vi "ForceBreakPt.vi"(2 "error in":errorcluster, 3 "Bd ID in":u8=1) -> (0 "error out":errorcluster, 1 "Bd ID Out":u8=1)   [LabVIEW 2022 SP3]
uses:
  <vilib>/Motion/FlexMotion/FunctionsVIs/MotionIO.llb/Set Breakpoint Output MOMO (8 axes).flx
  <vilib>/Motion/FlexMotion/CustomControls/CustomControls.llb/Mask (8 axes).flx
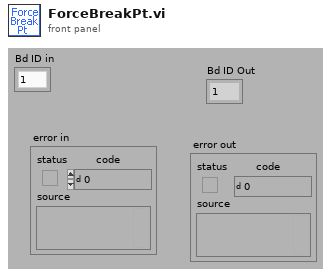
[diagram p1: front panel]
types:
  T1 = typedef "Mask (8 axes).flx" = cluster{"1":bool, "2":bool, "3":bool, "4":bool, "5":bool, "6":bool, "7":bool, "8":bool}
  T2 = typedef "Bd Id Out" = u8
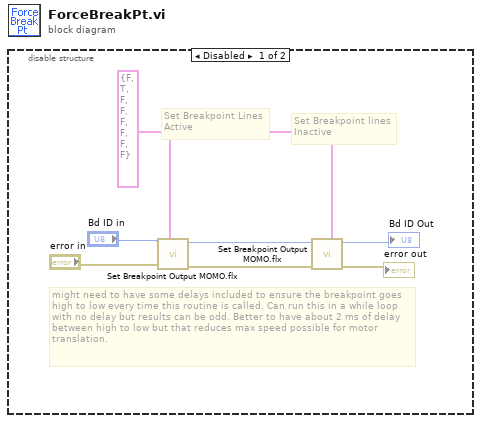
[diagram p0: block diagram]
diagram:
  n1 = disable-structure shown="Disabled" {
    frame Disabled {
      w1 = T1 {"1"=FALSE, "2"=TRUE, "3"=FALSE, "4"=FALSE, "5"=FALSE, "6"=FALSE, "7"=FALSE, "8"=FALSE} ("Must On (False)")
      # "might need to have some delays included to ensure the breakpoint goes high to low every time this routine is called. Can run this in a while loop with no delay but results can be odd. Better to have about 2 ms of delay between high to low but that reduces max speed possible for motor translation."
      # "Set Breakpoint Lines\nActive"
      # "Set Breakpoint lines\nInactive"
      n2 = call-poly <vilib>:"Set Breakpoint Output MOMO.flx"("Must On (False)"=w1, "error in (no error)"="error in", "Board ID"="Bd ID in") -> ("error out"=w6:errorcluster, "Bd ID Out"=w7:T2)  [unwired: 4 in, 1 out]
      n3 = call-poly <vilib>:"Set Breakpoint Output MOMO.flx"("Must Off (False)"=w1, "error in (no error)"=w6, "Board ID"=w7) -> ("error out"=→"error out":errorcluster, "Bd ID Out"=→"Bd ID Out":T2)  [unwired: 4 in, 1 out]
    }
    frame Enabled {
    }
  }
